vi "Get AI Data from local Daq Q.vi"(8 "error in":errorcluster, 11 "daqThread AI local Q":refnum<queue>) -> (0 "error out":errorcluster, 1 "timestamp":dbl, 2 "data":dbl[][](array[numeric]) format="%0.2f", 3 "daqThread AI local Q out":refnum<queue>, 5 "Q element":T1)   [LabVIEW 2017, in "DAQ.lvclass"]
doc: "Developed by Kevin Thompson\nkevin@thompsonengineering.net\n\nCopyright 2018-2020\nThompson Engineering, LLC"
uses:
  DAQ.lvclass
  TD local raw AI Data--cluster.ctl
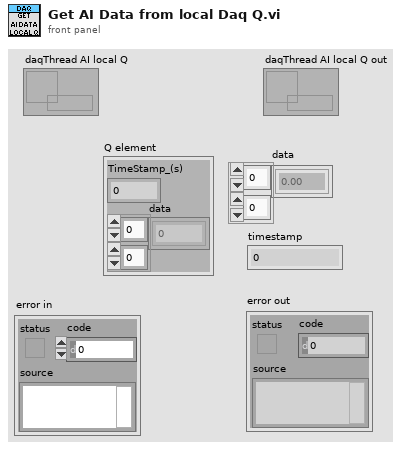
[diagram p1: front panel]
types:
  T1 = typedef "DAQ.lvclass/TD local raw AI Data--cluster.ctl" = cluster{"TimeStamp_(s)":dbl, "data":dbl[][]}
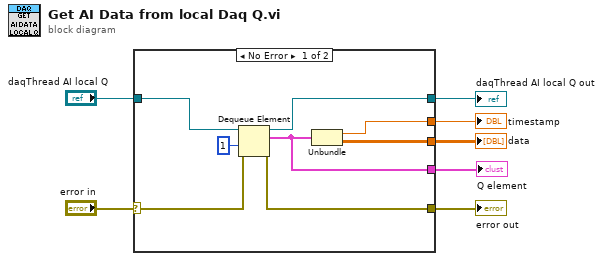
[diagram p0: block diagram]
diagram:
  n1 = case shown="No Error" "error in" {
    selector: "error in" -> [w9 w16]
    tunnel: "daqThread AI local Q" -> [w15 w17]
    tunnel: [w14 _] -> w6
    tunnel: [w13 _] -> w5
    tunnel: [w11 w16] -> w4
    tunnel: [w10 w17] -> w3
    tunnel: [w8 _] -> w1
    frame No Error {
      n2 = Dequeue Element(queue=w15, timeout in ms (-1)=1, error in (no error)=w9) -> (queue out=w10:refnum<queue>, element=w8:T1, error out=w11:errorcluster)  [unwired: 1 out]
      n3 = Unbundle(w8) -> ("TimeStamp_(s)"=w14:dbl, "data"=w13:dbl[][])
    }
    frame Error {
    }
  }
  "error out" <- w4
  "data" <- w5
  "timestamp" <- w6
  "daqThread AI local Q out" <- w3
  "Q element" <- w1
